vi "Lookup Group (Name).vi"(8 "error in (no error)":errorcluster, 10 "Group Name":string, 11 "Task Config in":refnum<class "Task Config.lvclass">) -> (0 "error out":errorcluster, 2 "Group Config":refnum<class "Group Config.lvclass">, 3 "Task Config out":refnum<class "Task Config.lvclass">)   [LabVIEW 2023, in "VolatusConfig.lvlib" / "Task Config.lvclass"]
uses:
  Task Config.lvclass
  Task Config.lvclass/Task Config.ctl
  VolatusConfig.lvlib
  Meta Type.ctl
  lv-cdm/CDM-Config/Config Filter/Config Lookup.lvclass
  VolatusConfigElement/VolatusConfigElement.lvclass
  C:/dev/volatus/mts-volatus-super/libs/lv-volatus/VolatusConfig/VolatusConfigElement/VolatusConfigElement.lvclass
  C:/dev/volatus/mts-volatus-super/libs/lv-volatus/VolatusConfig/Task/Task Config.lvclass
  Group/Group Config.lvclass
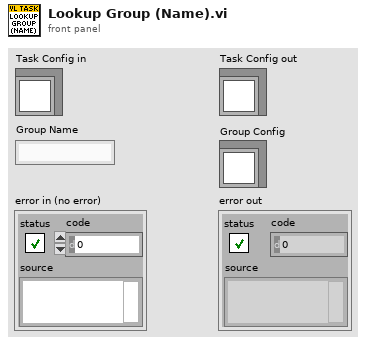
[diagram p1: front panel]
types:
  T1 = typedef "VolatusConfig.lvlib/Meta Type.ctl" = enum16{"UNKNOWN", "VL_System", "VL_Cluster", "VL_Node", "VL_Task", "VL_Group", "VL_Channel", "VL_Task_List", "VL_Scaling", "VL_Sensor", "VL_Sensor_List", "VL_Scale"}
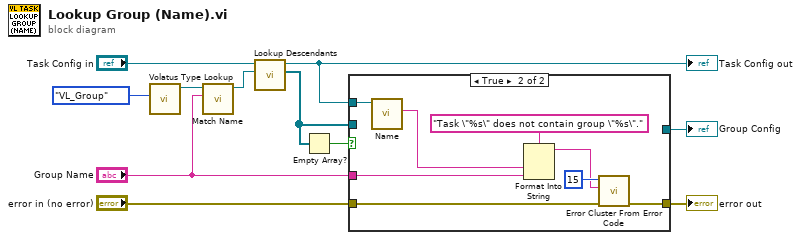
[diagram p0: block diagram]
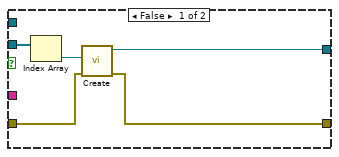
[diagram p2: hidden frame]
diagram:
  n1 = call "Volatus Type Lookup.vi"("Meta Type"=Meta_Type."VL_Group") -> ("Config Lookup out"=w9:refnum<class "Config Lookup.lvclass">)  [unwired: 9 in, 1 out]
  n2 = call "Match Name.vi"("Name"="Group Name", "Config Lookup (New)"=w9) -> ("Config Lookup out"=w8:refnum<class "Config Lookup.lvclass">)  [unwired: 8 in, 1 out]
  n3 = call "Lookup Descendants.vi"("Lookup"=w8, "VolatusConfigElement in"="Task Config in") -> ("Descendants"=w5:refnum<class "Config Element.lvclass">[], "VolatusConfigElement out"=w3:refnum<class "Task Config.lvclass">)  [unwired: 7 in, 1 out]
  "Task Config out" <- w3
  n4 = Empty Array?(array=w5) -> (empty?=w6:bool)
  n5 = case shown="True" w6 {
    tunnel: "error in (no error)" -> [w14 w24]
    tunnel: w5 -> [w16 _]
    tunnel: [w13 w23] -> w4
    tunnel: w3 -> [_ w22]
    tunnel: "Group Name" -> [_ w19]
    tunnel: [w12 _] -> w1
    frame False {
      n6 = Index Array(array=w16) -> (element=w15:refnum<class "Config Element.lvclass">)  [unwired: 1 in]
      n7 = call "Create.vi"("error in (no error)"=w14, "Element"=w15) -> ("error out"=w13:errorcluster, "Group out"=w12:refnum<class "Group Config.lvclass">)  [unwired: 8 in]
    }
    frame True {
      n8 = call "Name.vi"("VolatusConfigElement in"=w22) -> ("Name"=w17:string)  [unwired: 8 in, 2 out]
      n9 = Format Into String(format string="Task \"%s\" does not contain group \"%s\".", w17, w19) -> (resulting string=w18:string)  [unwired: 2 in, 1 out]
      n10 = call <vilib>:"Error Cluster From Error Code.vi"("error in (no error)"=w24, "error message (\"\")"=w18, "error code (0)"=15) -> ("error out"=w23:errorcluster)  [unwired: 6 in]
    }
  }
  "error out" <- w4
  "Group Config" <- w1
